vi "SEA_TRANSPARENCY_TESTING.vi"() -> ()   [LabVIEW 2019]
uses:
  Transparency target data.ctl
  <vilib>/Platform/TimedLoop/XDataNode/timing_clust.ctl
  <vilib>/Platform/TimedLoop/XDataNode/nitl_modes.ctl
  <vilib>/Platform/TimedLoop/XDataNode/wakeup.ctl
  <vilib>/FPGAPlugInAG/sbRIO-9627/niLvFpga_Open_sbRIO-9627.vi
  <vilib>/rvi/interface/common/dynamic/niFpgaDynamicAddResources.vi
  <vilib>/Utility/error.llb/Error Cluster From Error Code.vi
  <vilib>/rvi/errors/niLvFpgaAdjustHostInterfaceError.vi
  <vilib>/FPGAPlugInAG/Dynamic/niLvFpga_Close_Dynamic.vi
  <vilib>/rvi/interface/nirviOpenFPGA/nirviOpenFPGA.xnode
  FPGA Bitfiles/seafinalexperime_FPGATarget_SEALOWERLEVELPIC_AplcQzvwIw0.lvbitx
  SEA_LOWER_LEVEL_PI_CONTROL.vi
  <vilib>/platform/TimedLoop/XDataNode/XDataNode.xnode
  <vilib>/rvi/interface/nirviReadWriteControl/nirviReadWriteControl.xnode
  <vilib>/rvi/interface/nirviCloseFPGA/nirviCloseFPGA.xnode
  <vilib>/Platform/TimedLoop/XDataNode/XDNodeRunTimeDep.lvlib
  NiFpgaLv.dll
  <vilib>/rvi/interface/Simulation/niFpgaSimulationCallBeginRW.vi
panel:
  in  "Cluster":T1
  out "Torque":cluster{"x":sgl, sgl}(graph)
  in  "Ki torque control":sgl
  in  "Position Reset":bool
  in  "torque control lower limit":sgl
  in  "torque control upper limit":sgl
  in  "Kp torque control":sgl
  out "Position integrator o/p":sgl
  in  "Ki integrator":sgl
  out "pos_ctrl_ip":sgl
  out "Transparency current":T2(graph)
  out "Transparency position":T3(graph)
  out "Finished late count":u32
  in  "transparency current lower limit":sgl
  in  "transparency current upper limit":sgl
  in  "Kp position":sgl
  in  "Amplitude":sgl
  in  "frequency":sgl
  in  "transparency motor Lower bound":sgl
  in  "transparency motor Upper bound":sgl
  in  "transparency motor Ki current control":sgl
  in  "transparency motor Kp current control":sgl
  in  "transparency Current Offset":sgl
  in  "Position Reset transparency side":bool
  in  "Position Reset joint side":bool
  in  "Lower bound":sgl
  in  "Upper bound":sgl
  in  "Ki current control":sgl
  in  "Kp current control":sgl
  in  "Current Offset":sgl
  in  "stop":bool
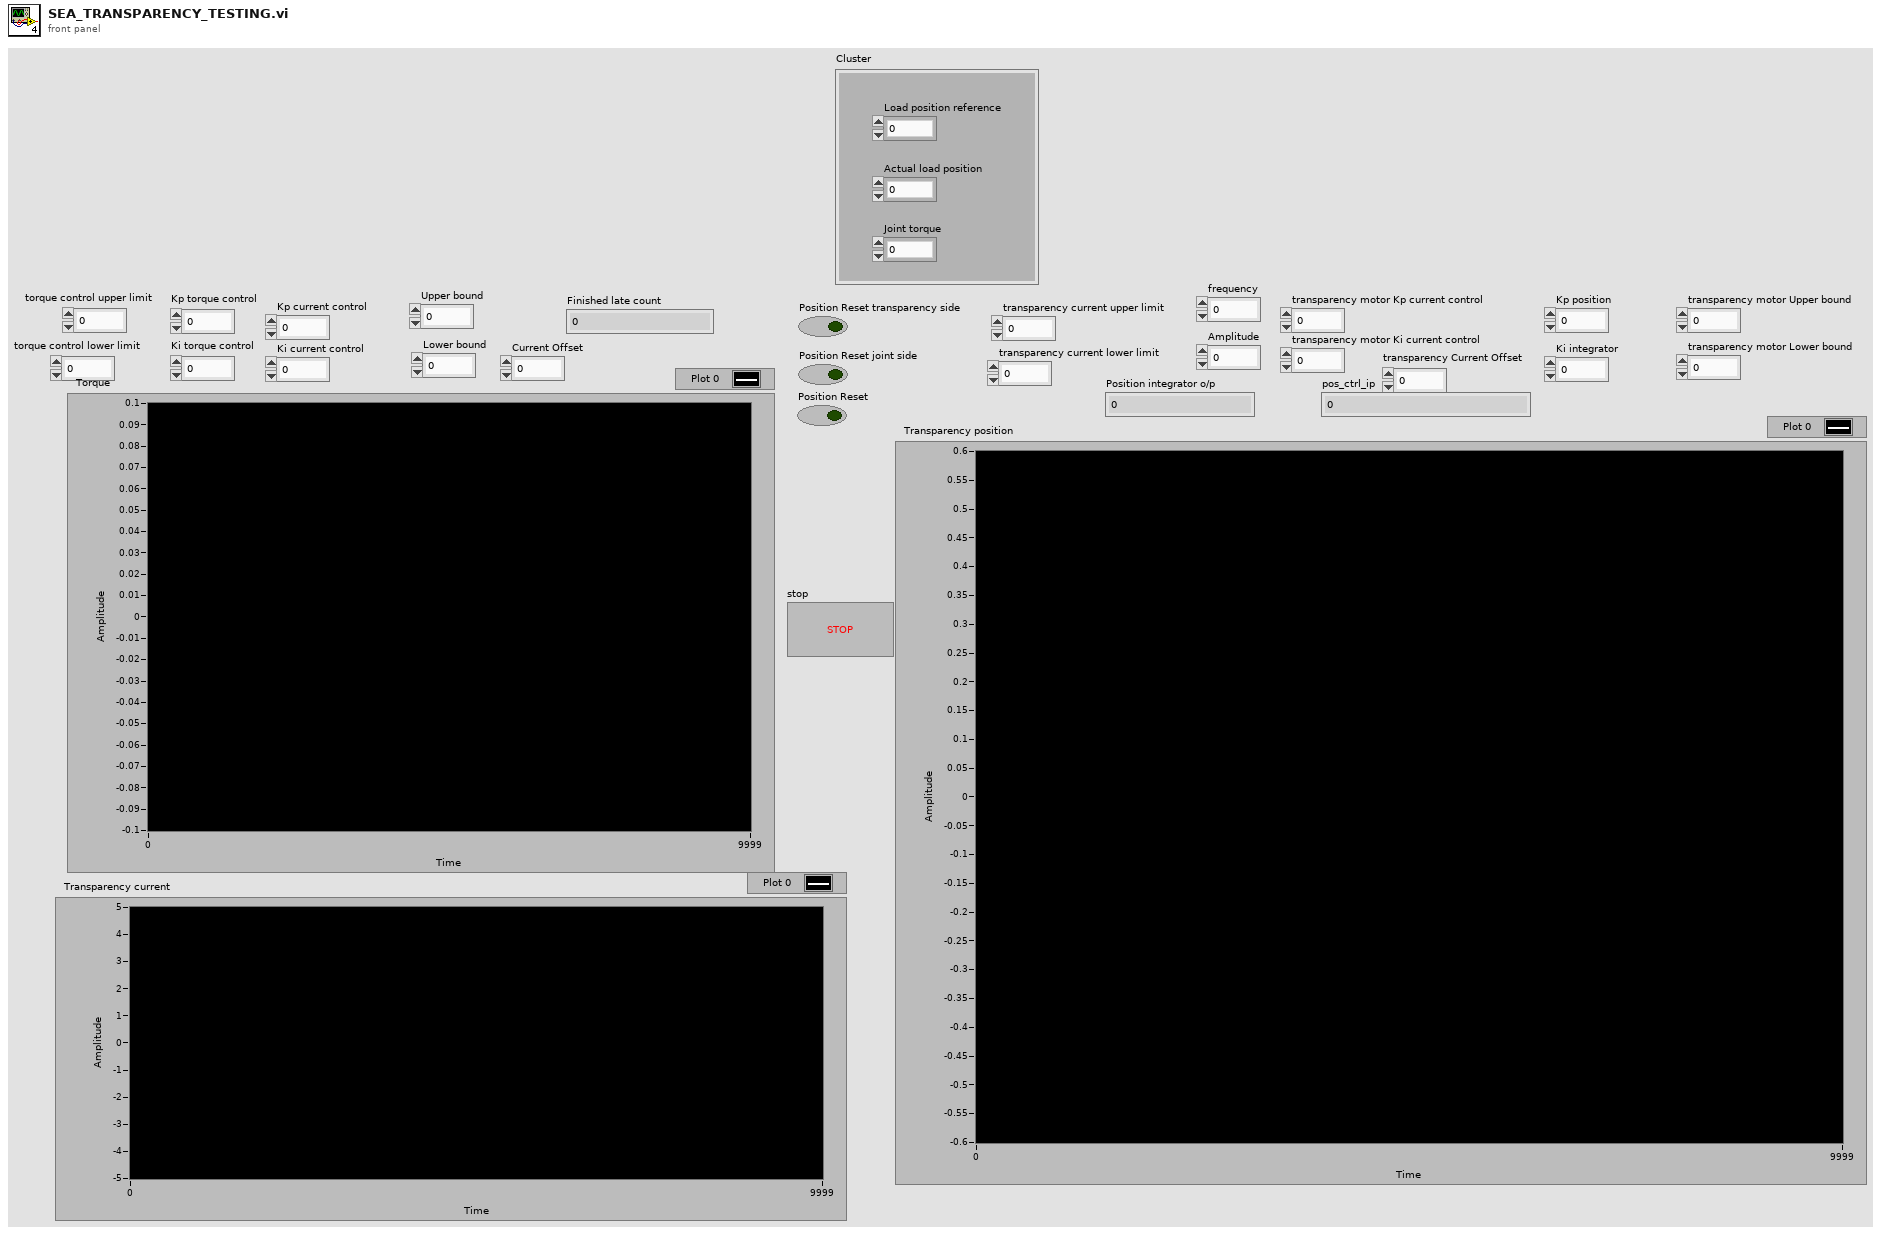
[diagram p1: front panel]
types:
  T1 = typedef "Transparency target data.ctl" = cluster{"Load position reference":sgl, "Actual load position":sgl, "Joint torque":sgl}
  T2 = cluster{sgl, "transparency filtered current":sgl}
  T3 = cluster{sgl, "Position(Radians) transparency motor side":sgl}
  T4 = typedef "XDNodeRunTimeDep.lvlib/timing_clust.ctl" = cluster{"Expected End [f-1]":u64, "Actual End [f-1]":u64, "Finished Late? [f-1]":bool, "Expected End [i-1]":u64, "Actual End [i-1]":u64, "Finished Late? [i-1]":bool, "Expected Start [i]":u64, "Actual Start [i]":u64, "Expected Start [f]":u64, "Actual Start [f]":u64, "Source Name":string, "Structure Name":string, "Period":i64, "Deadline":i64, "Offset":i64, "Start":i64, "Priority":i32, "Timeout":i32, "Mode":T5, "Wakeup Reason":T6, "Error":errorcluster, "Source Type":string, "Secondary Source Type":string, "Global End Time":u64, "Global Start Time":u64, "Frame Duration":u64, "Iteration Duration":u64, "Assigned CPU":i32, "I/O Scan Engine Mode":u32}
  T5 = typedef "XDNodeRunTimeDep.lvlib/nitl_modes.ctl" = enum32{"No Change", "Process missed periods, maintain original phase", "Discard missed periods, maintain original phase", "Process missed periods, ignore original phase", "Discard missed periods, ignore original phase"}
  T6 = typedef "XDNodeRunTimeDep.lvlib/wakeup.ctl" = enum32{"Normal", "Aborted", "Asynchronous wakeup", "Timing source error", "Timed loop error", "Timeout"}
  T7 = cluster{"transparency current upper limit":sgl, "transparency filtered current":sgl}
  T8 = enum16{"open", "open or create", "create or replace", "create", "open (read-only)"}
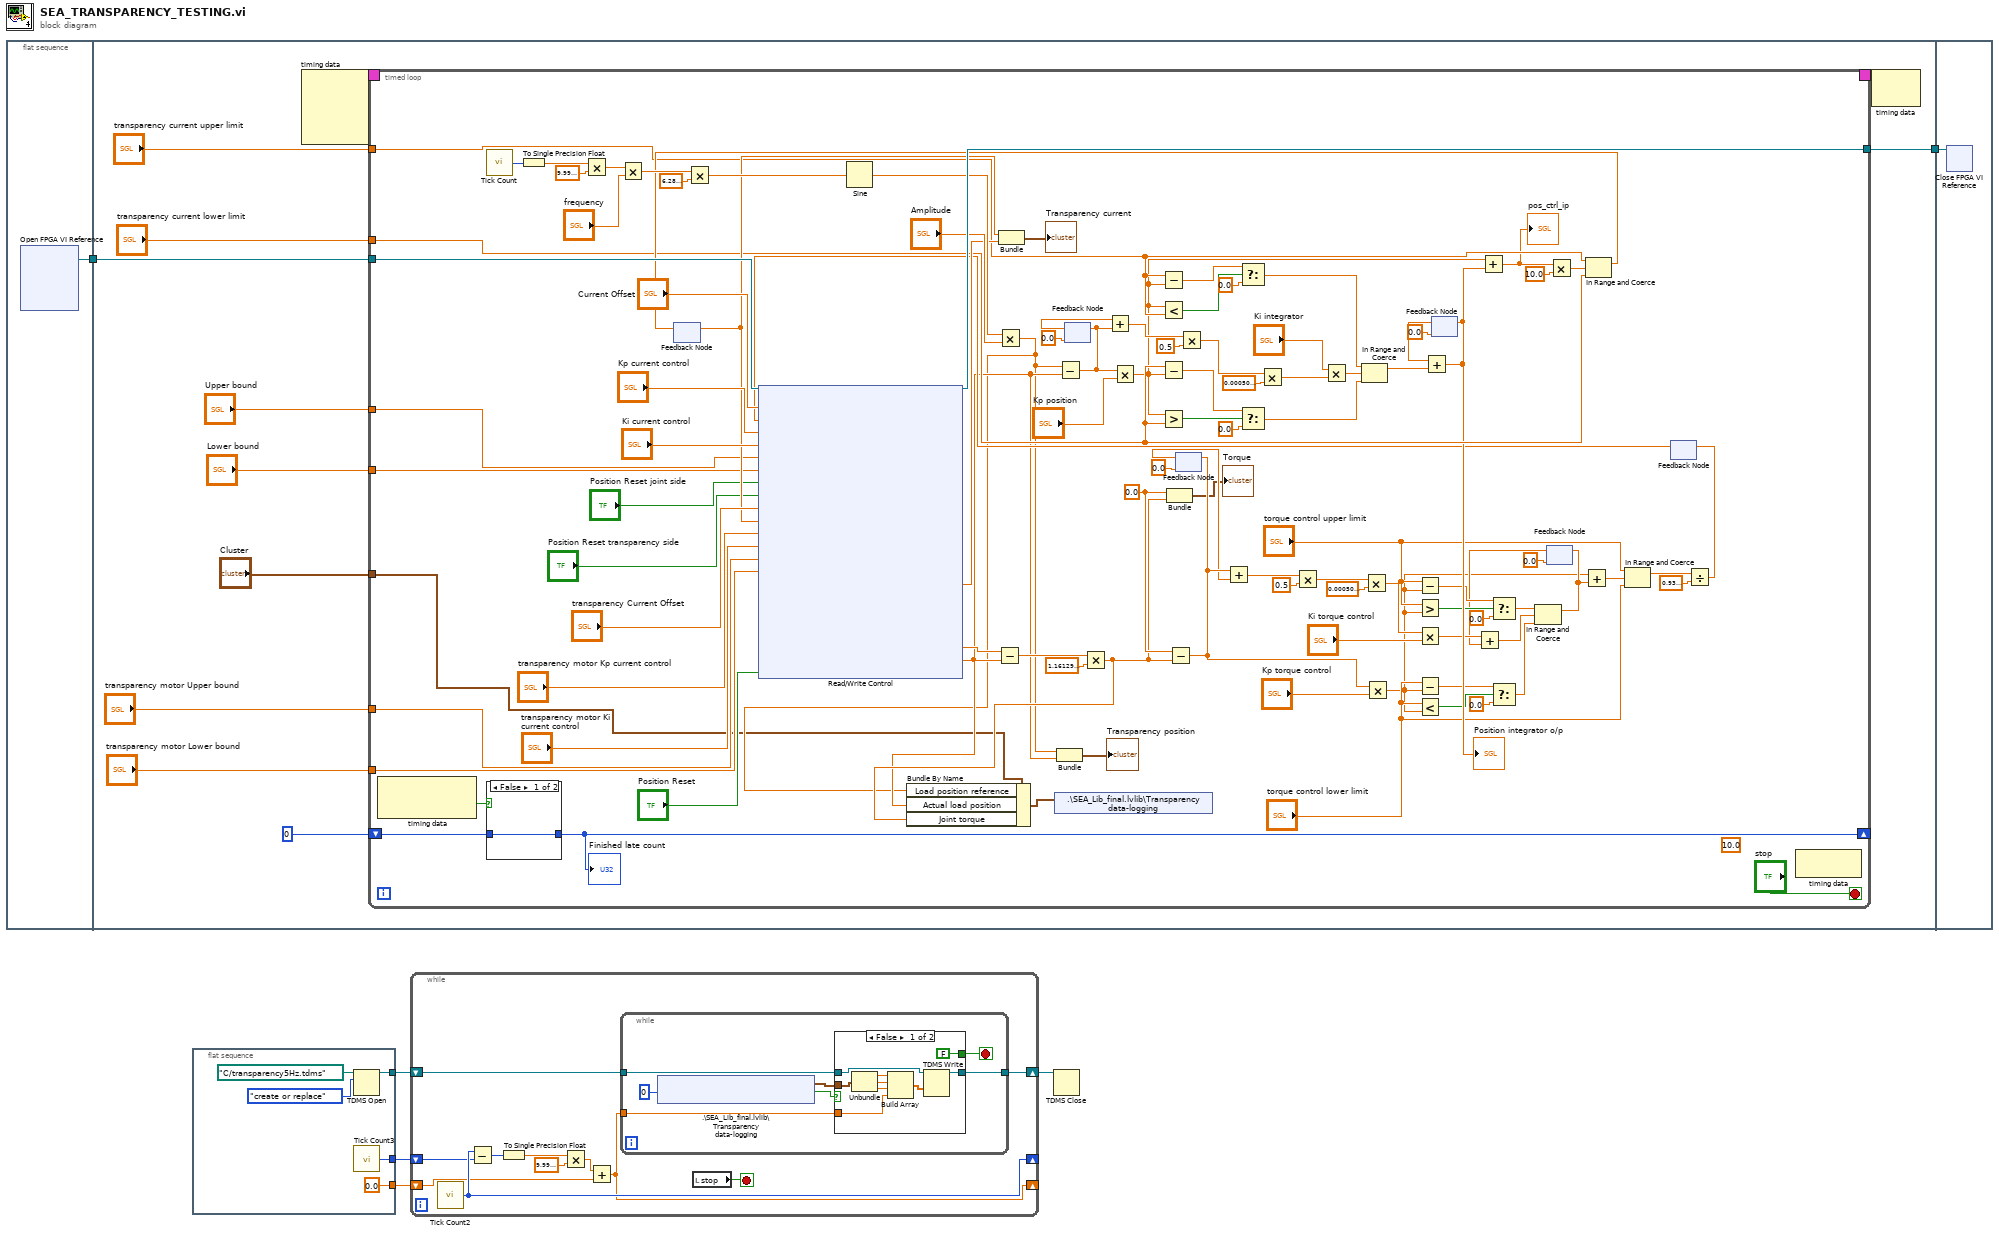
[diagram p0: block diagram]
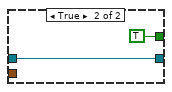
[diagram p2: hidden frame]
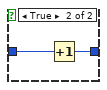
[diagram p3: hidden frame]
diagram:
  n1 = flat-sequence {
    tunnel: [w7] -> w6
    tunnel: w6 -> [w17]
    tunnel: [w16] -> w5
    tunnel: w5 -> [w132]
    frame #0 {
      n2 = xnode "Open FPGA VI Reference"() -> ("FPGA VI Reference Out"=w7:refnum<k20>)  [unwired: 2 in, 1 out]
    }
    frame #1 {
      n3 = node-c288() -> (w19:T4)  [unwired: 4 in]
      n4 = timed-loop {
        timing: w19 -> [_]
        timing-out: [_] -> w18
        tunnel: w17 -> [w122]
        tunnel: [w121] -> w16
        tunnel: "transparency motor Upper bound" -> [w101]
        tunnel: "transparency motor Lower bound" -> [w100]
        tunnel: "Upper bound" -> [w99]
        tunnel: "Lower bound" -> [w98]
        tunnel: "transparency current lower limit" -> [w85]
        tunnel: "transparency current upper limit" -> [w88]
        shift-right: [w95] -> _
        shift-left: u32 0 -> [w96]
        tunnel: "Cluster" -> [w20]
        stop <- "stop" stop-if-true
        w26 = sgl 0.0 ("x")
        (unwired) sgl 10.0 ("y")
        n5 = node-c288() -> (w97:bool)  [unwired: 1 in, 1 out]
        n6 = call "Tick Count"() -> ("Tick Count(uSec)"=w105:u32)
        n7 = case shown="False" w97 {
          tunnel: w96 -> [w124 w126]
          tunnel: [w124 w125] -> w95
          frame False {
          }
          frame True {
            n8 = Increment(x=w126) -> (x+1=w125:u32)
          }
        }
        "Finished late count" <- w95
        n9 = To Single Precision Float(number=w105) -> (single precision float=w114:sgl)
        n10 = Multiply(x=w114, y=sgl 1e-06) -> (x*y=w112:sgl)
        n11 = Multiply(x=w112, y="frequency") -> (x*y=w110:sgl)
        n12 = feedback #1() -> (w102:sgl)  [unwired: 1 in]
        n13 = Multiply(x=w110, y=sgl 6.28) -> (x*y=w108:sgl)
        n14 = Sine(x=w108) -> (sin(x)=w107:sgl)
        n15 = Multiply(x=w107, y="Amplitude") -> (x*y=w22:sgl)
        n16 = feedback #2(sgl 0.0) -> (w80:sgl)
        n17 = feedback #3(sgl 0.0) -> (w42:sgl)
        n18 = feedback #4(sgl 0.0) -> (w68:sgl)
        n19 = feedback #5(sgl 0.0) -> (w33:sgl)
        n20 = feedback #6() -> (w55:sgl)  [unwired: 1 in]
        n21 = xnode "Read/Write Control"("FPGA VI Reference In"=w122, "Current Offset"="Current Offset", "Reference"=w55, "Kp current control"="Kp current control", "Ki current control"="Ki current control", "Upper bound"=w99, "Lower bound"=w98, "Position Reset joint side"="Position Reset joint side", "Position Reset transparency side"="Position Reset transparency side", "transparency Current Offset"="transparency Current Offset", "transparency reference"=w102, "transparency motor Kp current control"="transparency motor Kp current control", "transparency motor Ki current control"="transparency motor Ki current control", "transparency motor Upper bound"=w101, "transparency motor Lower bound"=w100, "Position Reset"="Position Reset") -> ("FPGA VI Reference Out"=w121:refnum<k20>, "transparency filtered current"=w103:sgl, "Position(Radians) motor side"=w61:sgl, "Position(Radians) joint side"=w23:sgl)  [unwired: 1 in, 5 out]
        n22 = Subtract(x=w61, y=w23) -> (x-y=w44:sgl)
        n23 = Bundle("transparency current upper limit"=w102, "transparency filtered current"=w103) -> (→"Transparency current":T7)  [unwired: 1 in]
        n24 = Bundle(w22, "Position(Radians) joint side"=w23) -> (→"Transparency position":cluster{sgl, "Position(Radians) joint side":sgl})  [unwired: 1 in]
        n25 = Subtract(x=w22, y=w23) -> (x-y=w79:sgl)
        n26 = feedback-in #2(w79) -> ()
        n27 = Multiply(x=w44, y=sgl 1.1613) -> (x*y=w24:sgl)
        n28 = Bundle By Name(cluster=w20, "Load position reference"=w22, "Actual load position"=w23, "Joint torque"=w24) -> (w21:T1)
        n29 = shared-variable ".\\SEA_Lib_final.lvlib\\Transparency data-logging"(w21) -> ()  [unwired: 1 in, 1 out]
        n30 = Add(x=w80, y=w79) -> (x+y=w78:sgl)
        n31 = Multiply(x=w79, y="Kp position") -> (x*y=w65:sgl)
        n32 = Subtract(x=w88, y=w65) -> (x-y=w86:sgl)
        n33 = Less?(x=w65, y=w88) -> (x < y?=w89:bool)
        n34 = Subtract(x=w85, y=w65) -> (x-y=w84:sgl)
        n35 = Greater?(x=w65, y=w85) -> (0:w87:bool)
        n36 = Bundle("x"=w26, w24) -> (→"Torque":cluster{"x":sgl, sgl})  [unwired: 1 in]
        n37 = Subtract(x=w26, y=w24) -> (x-y=w43:sgl)
        n38 = feedback-in #3(w43) -> ()
        n39 = Multiply(x=w78, y=sgl 0.5) -> (x*y=w76:sgl)
        n40 = Add(x=w43, y=w42) -> (x+y=w41:sgl)
        n41 = Select(t=w86, s=w89, f=sgl 0.0) -> (s? t:f=w72:sgl)
        n42 = Select(t=w84, s=w87, f=sgl 0.0) -> (s? t:f=w71:sgl)
        n43 = Multiply(x=w76, y=sgl 0.0005) -> (x*y=w74:sgl)
        n44 = Multiply(x=w41, y=sgl 0.5) -> (x*y=w39:sgl)
        n45 = Multiply(x="Ki integrator", y=w74) -> (x*y=w70:sgl)
        n46 = In Range and Coerce(upper limit=w72, x=w70, lower limit=w71) -> (coerced(x)=w67:sgl)  [unwired: 1 out]
        n47 = Multiply(x=w39, y=sgl 0.0005) -> (x*y=w37:sgl)
        n48 = Multiply(x=w43, y="Kp torque control") -> (x*y=w28:sgl)
        n49 = Subtract(x="torque control upper limit", y=w28) -> (x-y=w51:sgl)
        n50 = Greater?(x="torque control upper limit", y=w28) -> (0:w53:bool)
        n51 = Multiply(x=w37, y="Ki torque control") -> (x*y=w34:sgl)
        n52 = Subtract(x="torque control lower limit", y=w28) -> (x-y=w47:sgl)
        n53 = Less?(x="torque control lower limit", y=w28) -> (x < y?=w49:bool)
        n54 = Add(x=w68, y=w67) -> (x+y=w66:sgl)
        "Position integrator o/p" <- w66
        n55 = feedback-in #4(w66) -> ()
        n56 = Add(x=w34, y=w33) -> (x+y=w30:sgl)
        n57 = Add(x=w65, y=w66) -> (x+y=w62:sgl)
        "pos_ctrl_ip" <- w62
        n58 = Select(t=w51, s=w53, f=sgl 0.0) -> (s? t:f=w32:sgl)
        n59 = Select(t=w47, s=w49, f=sgl 0.0) -> (s? t:f=w31:sgl)
        n60 = In Range and Coerce(upper limit=w32, x=w30, lower limit=w31) -> (coerced(x)=w29:sgl)  [unwired: 1 out]
        n61 = feedback-in #5(w29) -> ()
        n62 = Multiply(x=w62, y=sgl 10.0) -> (x*y=w63:sgl)
        n63 = Add(x=w28, y=w29) -> (x+y=w27:sgl)
        n64 = In Range and Coerce(upper limit=w88, x=w63, lower limit=w85) -> (coerced(x)=w92:sgl)  [unwired: 1 out]
        n65 = feedback-in #1(w92) -> ()
        n66 = In Range and Coerce(upper limit="torque control upper limit", x=w27, lower limit="torque control lower limit") -> (coerced(x)=w58:sgl)  [unwired: 1 out]
        n67 = Divide(x=w58, y=sgl 0.94) -> (x/y=w56:sgl)
        n68 = feedback-in #6(w56) -> ()
        n69 = node-c288() -> ()  [unwired: 1 in, 1 out]
      }
      n70 = node-c288(w18) -> ()  [unwired: 1 out]
    }
    frame #2 {
      n71 = xnode "Close FPGA VI Reference"("FPGA VI Reference In"=w132) -> ()  [unwired: 1 in, 1 out]
    }
  }
  n72 = flat-sequence {
    tunnel: [w135] -> w4
    tunnel: [w134] -> w2
    tunnel: [sgl 0.0] -> w1
    frame #0 {
      n73 = TDMS Open(10:T8."create or replace" ("operation (0:open)"), 11:path "C:/transparency5Hz.tdms" ("file path")) -> (3:w135:refnum<k34>)  [unwired: 5 in, 1 out]
      n74 = call "Tick Count3"() -> ("Tick Count(uSec)"=w134:u32)
    }
  }
  n75 = while {
    shift-right: [w147] -> w3
    shift-left: w4 -> [w148]
    shift-right: [w146] -> _
    shift-left: w2 -> [w145]
    shift-right: [w139] -> _
    shift-left: w1 -> [w140]
    stop <- w138 stop-if-true
    n76 = call "Tick Count2"() -> ("Tick Count(uSec)"=w146:u32)
    n77 = Subtract(x=w146, y=w145) -> (x-y=w144:u32)
    n78 = To Single Precision Float(number=w144) -> (single precision float=w143:sgl)
    n79 = Multiply(x=w143, y=sgl 1e-06) -> (x*y=w142:sgl)
    n80 = Add(x=w142, y=w140) -> (x+y=w139:sgl)
    n81 = while {
      tunnel: w148 -> [w152]
      tunnel: [w150] -> w147
      tunnel: w139 -> [w149]
      stop <- w153 stop-if-true
      n82 = shared-variable ".\\SEA_Lib_final.lvlib\\Transparency data-logging"(0 ("ms timeout (0)")) -> (w151:T1, w154:bool)  [unwired: 1 in, 1 out]
      n83 = case shown="False" w154 {
        tunnel: [FALSE TRUE] -> w153
        tunnel: w152 -> [w164 w165]
        tunnel: w151 -> [w163 _]
        tunnel: [w158 w165] -> w150
        tunnel: w149 -> [w156 _]
        frame False {
          n84 = Unbundle(w163) -> ("Load position reference"=w162:sgl, "Actual load position"=w161:sgl, "Joint torque"=w160:sgl)
          n85 = Build Array(w162, w161, w160, w156) -> (w159:sgl[])
          n86 = TDMS Write(0:w164, 9:w159) -> (4:w158:refnum<k34>)  [unwired: 4 in, 3 out]
        }
        frame True {
        }
      }
    }
    n87 = local read "stop"() -> (w138:bool)
  }
  n88 = TDMS Close(11:w3) -> ()  [unwired: 1 in, 2 out]
